vi "Write STAR.vi"(8 "error in (no error)":errorcluster, 10 "STAR":refnum<vi>, 11 "Star in":refnum<class "Star.lvclass">) -> (0 "error out":errorcluster, 3 "Star out":refnum<class "Star.lvclass">)   [LabVIEW 2021, in "Star.lvclass"]
uses:
  Star.lvclass
  Star.lvclass/Star.ctl
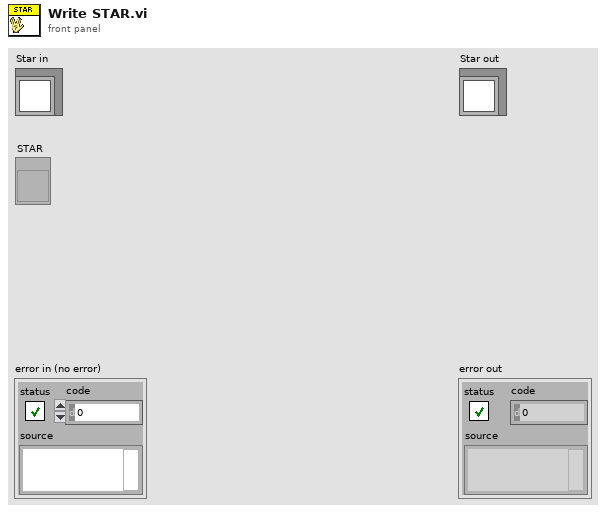
[diagram p1: front panel]
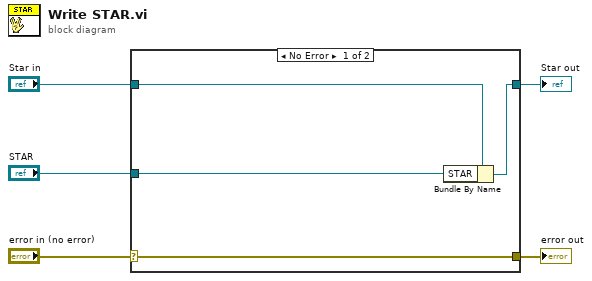
[diagram p0: block diagram]
diagram:
  n1 = case shown="No Error" "error in (no error)" {
    selector: "error in (no error)" -> [w9 w10]
    tunnel: [w9 w10] -> w4
    tunnel: [w7 w11] -> w2
    tunnel: "Star in" -> [w8 w11]
    tunnel: "STAR" -> [w6 _]
    frame No Error {
      n2 = Bundle By Name(cluster=w8, "STAR"=w6) -> (w7:refnum<class "Star.lvclass">)
    }
    frame Error {
    }
  }
  "error out" <- w4
  "Star out" <- w2
